vi "M13_Flywheel_Hardware.vi"   [LabVIEW 2019]
uses:
  <vilib>/Rock Robotics/WPI/ThirdParty/REV Robotics/SPARK MAX/Typedef/Spark MAX Control Type.ctl
  Flywheel/Flywheel_Globals.vi
  Utility_VIs/Basic_Motor_Modes.ctl
types:
  T1 = typedef "WPI_MotorControlDeviceRef.ctl" = cluster{"DeviceStatus":errorcluster, "Type":T2, "PWM":cluster{"PWM Channel":T3, "DeadBand":T4}, "CAN":cluster{"Device Number":u8, "SetOutput VI Ref":variant, "GetOutput VI Ref":variant, "Enable VI Ref":variant, "Disable VI Ref":variant, "Data":variant}, "Invert":bool, "DIO PWM":cluster{"PWM \"Enable\" Channel":T3, "DIOChannel":T5, "PWM Rate":dbl}}
  T2 = typedef "WPI_MotorControlType.ctl" = enum16{"PWM", "CAN", "DIO PWM"}
  T3 = typedef "FPGA_DIOPWMChannel.ctl" = enum8{"PWM 0", "PWM 1", "PWM 2", "PWM 3", "PWM 4", "PWM 5", "PWM 6", "PWM 7", "PWM 8", "PWM 9", "PWM MXP 0", "PWM MXP 1", "PWM MXP 2", "PWM MXP 3", "PWM MXP 4", "PWM MXP 5", "PWM MXP 6", "PWM MXP 7", "PWM MXP 8", "PWM MXP 9", "Invalid"}
  T4 = typedef "WPI_PWMDeadband.ctl" = cluster{"Name":string, "maxPositivePwm":i32, "minPositivePwm":i32, "centerPwm":i32, "maxNegativePwm":i32, "minNegativePwm":i32, "angularRange":u16}
  T5 = typedef "FPGA_DIOChannel.ctl" = enum8{"DIO 0", "DIO 1", "DIO 2", "DIO 3", "DIO 4", "DIO 5", "DIO 6", "DIO 7", "DIO 8", "DIO 9", "DIO MXP 0", "DIO MXP 1", "DIO MXP 2", "DIO MXP 3", "DIO MXP 4", "DIO MXP 5", "DIO MXP 6", "DIO MXP 7", "DIO MXP 8", "DIO MXP 9", "DIO MXP 10", "DIO MXP 11", "DIO MXP 12", "DIO MXP 13", "DIO MXP 14", "DIO MXP 15", "SPI Port CS1", "SPI Port CS2", "SPI Port CS3", "SPI Port MISO", "SPI Port MOSI", "Invalid"}
  T6 = typedef "Spark MAX Control Type.ctl" = enum16{"Percent VBus", "Voltage", "Velocity", "Position", "Smart Motion", "Current", "Smart Velocity"}
  T7 = typedef "Basic_Motor_Modes.ctl" = enum16{"Percent_Voltage", "Speed_Control", "Position_Control", "Current"}
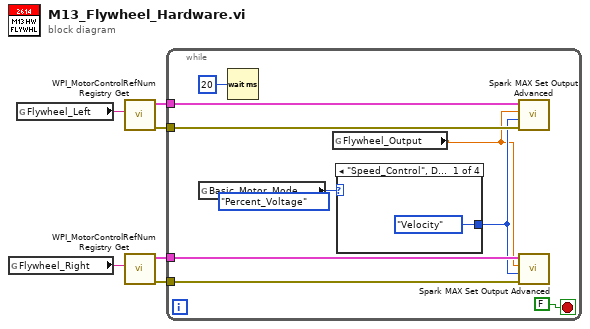
[diagram p0: block diagram]
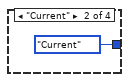
[diagram p2: hidden frame]
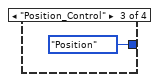
[diagram p3: hidden frame]
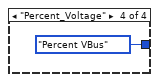
[diagram p4: hidden frame]
diagram:
  n1 = global read "Flywheel_Globals.vi" "Flywheel_Right"() -> (w1:string)
  n2 = global read "Flywheel_Globals.vi" "Flywheel_Left"() -> (w2:string)
  n3 = call <vilib>:"WPI_MotorControlRefNum Registry Get.vi"("refnum name"=w2) -> ("error out"=w4:errorcluster, "MotorControlDevRef"=w6:T1)  [unwired: 9 in]
  n4 = call <vilib>:"WPI_MotorControlRefNum Registry Get.vi"("refnum name"=w1) -> ("error out"=w3:errorcluster, "MotorControlDevRef"=w5:T1)  [unwired: 9 in]
  n5 = while {
    tunnel: w6 -> [w13]
    tunnel: w5 -> [w12]
    tunnel: w4 -> [w11]
    tunnel: w3 -> [w10]
    stop <- FALSE stop-if-true
    (unwired) Basic_Motor_Modes."Percent_Voltage" ("Motor_Mode")
    n6 = global read "Flywheel_Globals.vi" "Basic_Motor_Mode"() -> (w8:T7)
    n7 = Wait (ms)(milliseconds to wait=u32 20) -> ()  [unwired: 1 out]
    n8 = global read "Flywheel_Globals.vi" "Flywheel_Output"() -> (w7:dbl)
    n9 = case shown="\"Speed_Control\", Default" w8 {
      tunnel: [Spark_MAX_Control_Type."Velocity" ("Control Mode") Spark_MAX_Control_Type."Current" ("Control Mode") Spark_MAX_Control_Type."Position" ("Control Mode") Spark_MAX_Control_Type."Percent VBus" ("Control Mode")] -> w9
      frame "Speed_Control", Default {
      }
      frame "Current" {
      }
      frame "Position_Control" {
      }
      frame "Percent_Voltage" {
      }
    }
    n10 = call <vilib>:"Spark MAX Set Output Advanced.vi"("error in (no error)"=w11, "Control Mode"=w9, "Setpoint"=w7, "MotorControlDevRef"=w13) -> ()  [unwired: 6 in, 2 out]
    n11 = call <vilib>:"Spark MAX Set Output Advanced.vi"("error in (no error)"=w10, "Control Mode"=w9, "Setpoint"=w7, "MotorControlDevRef"=w12) -> ()  [unwired: 6 in, 2 out]
  }
